vi "Create Staffs Map.vi"(11 "error in (no error)":errorcluster) -> (4 "Staffs List Map":map{string, T1}(c390), 15 "error out":errorcluster)   [LabVIEW 2023, in "File Data Manager.lvlib" / "File Data Manager.lvclass"]
uses:
  File Data Manager.lvclass
  Central Data Manager/Central Data Manager/Staff Details.ctl
  Central Data Manager/Central Data Manager/Staff Designation.ctl
  Central Data Manager/Central Data Manager/Staff Attendance.ctl
  c16a2279-ec5c-4c78-9d40-d4802565a870.vi
  2f043f59-072d-4791-84bb-8087a6f89dc8.vi
  <vilib>/Utility/file.llb/Read Delimited Spreadsheet (string).vi
  Utilities/Utilities.lvlib
  Central Data Manager/Central Data Manager/Central Data Manager.lvclass
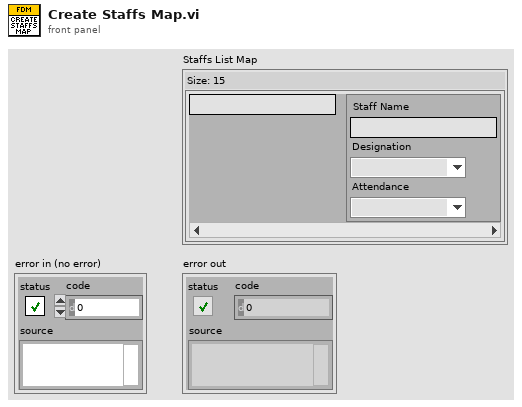
[diagram p1: front panel]
types:
  T1 = typedef "Central Data Manager.lvlib/Central Data Manager.lvclass/Staff Details.ctl" = cluster{"Staff Name":string, "Designation":T2, "Attendance":T3}
  T2 = typedef "Central Data Manager.lvlib/Central Data Manager.lvclass/Staff Designation.ctl" = enum16{"Manager", "Receptionist", "Chef", "Waiter", "Room Service"}
  T3 = typedef "Central Data Manager.lvlib/Central Data Manager.lvclass/Staff Attendance.ctl" = enum16{"Present", "Absent"}
  T4 = typedef "Hotel Management Tool Model.lvlib/Hotel Management Tool Model.lvclass/Database File Paths.ctl" = cluster{"Food Menu File Path":path, "Guests Histroy File Path":path, "Room Size File Path":path, "Rooms List File Path":path, "Rooms Service Allocation File Path":path, "Staff List File Path":path}
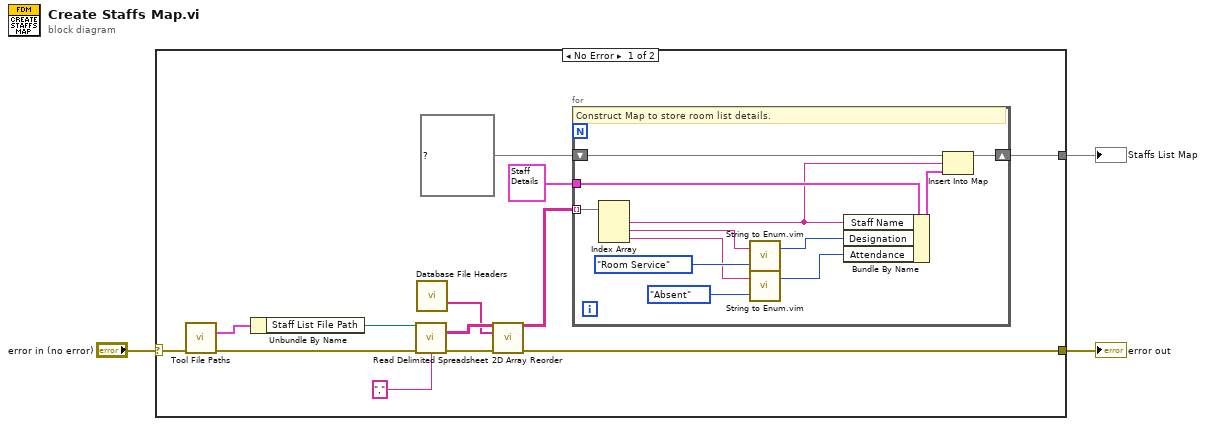
[diagram p0: block diagram]
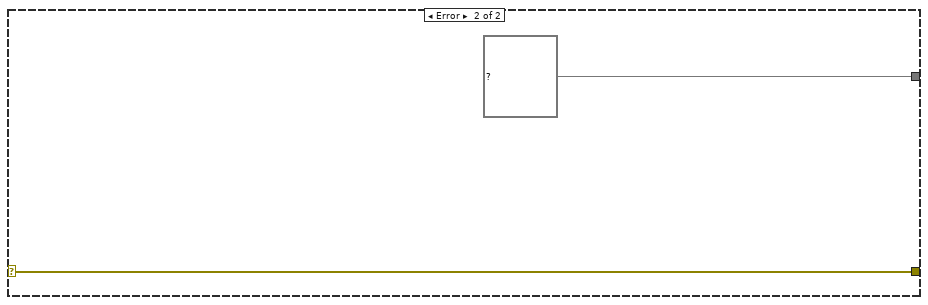
[diagram p2: hidden frame]
diagram:
  n1 = case shown="No Error" "error in (no error)" {
    selector: "error in (no error)" -> [w10 w30]
    tunnel: [w8 w30] -> w2
    tunnel: [w7 map{string, T1} {} ("Rooms List")] -> w1
    frame No Error {
      n2 = call "Tool File Paths.vi"("error in (no error)"=w10) -> ("Database File Paths"=w16:T4, "error out"=w15:errorcluster)  [unwired: 12 in, 1 out]
      n3 = Unbundle By Name(w16) -> ("Staff List File Path"=w14:path)
      n4 = call-poly <vilib>:"Read Delimited Spreadsheet.vi"("file path (dialog if empty)"=w14, "error in (no error)"=w15, "delimiter (\\t)"="," ("delimiter (\\t)")) -> ("all rows"=w11:string[][], "error out"=w12:errorcluster)  [unwired: 7 in, 4 out]
      n5 = call "Database File Headers.vi"() -> ("Staffs List Headers"=w5:string[])  [unwired: 12 in, 3 out]
      n6 = call "2D Array Reorder.vi"("2D Array Data witjh Header"=w11, "Header Order"=w5, "error in (no error)"=w12) -> ("Reordered Data without Header"=w9:string[][], "error out"=w8:errorcluster)  [unwired: 11 in]
      n7 = for {
        tunnel: w9 -> [w25] mode=indexing
        shift-right: [w27] -> w7
        shift-left: map{string, T1} {} ("Staffs List Map") -> [w28]
        tunnel: T1 {"Staff Name"="", "Designation"=enum."Manager", "Attendance"=enum."Present"} ("Guest Details") -> [w26]
        # "Construct Map to store room list details."
        n8 = Index Array(array=w25) -> (element #1=w24:string, element #2=w22:string, element #3=w18:string)  [unwired: 3 in]
        n9 = call "String to Enum.vim"("Enum Type"=Staff_Designation."Room Service" ("Designation"), "Input String"=w22) -> ("Output"=w20:T2)
        n10 = call "String to Enum.vim"("Enum Type"=Staff_Attendance."Absent" ("Attendance"), "Input String"=w18) -> ("Output"=w17:T3)
        n11 = Bundle By Name(cluster=w26, "Staff Name"=w24, "Designation"=w20, "Attendance"=w17) -> (w23:T1)
        n12 = Insert Into Map(map in=w28, key=w24, value=w23) -> (map out=w27:map{string, T1})  [unwired: 2 out]
      }
    }
    frame Error {
    }
  }
  "error out" <- w2
  "Staffs List Map" <- w1
